vi "Packets_per_burst.vi"(8 "Message bits per packet":i32=128, 9 "Bits per sample":i32=16, 10 "Audio record time/delay (ms)":i32=200, 11 "Audio sample rate (Fs)":i32=6000) -> (3 "Packets per burst":i32)   [LabVIEW 2014]
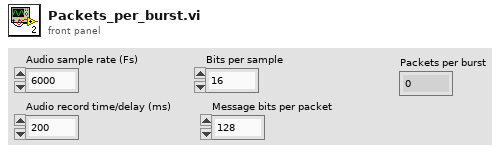
[diagram p1: front panel]
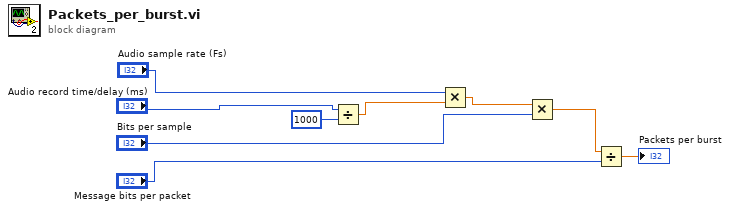
[diagram p0: block diagram]
diagram:
  n1 = Divide(x="Audio record time/delay (ms)", y=1000) -> (x/y=w6:dbl)
  n2 = Multiply(x="Audio sample rate (Fs)", y=w6) -> (x*y=w5:dbl)
  n3 = Multiply(x=w5, y="Bits per sample") -> (x*y=w2:dbl)
  n4 = Divide(x=w2, y="Message bits per packet") -> (x/y=→"Packets per burst":dbl)
